vi "Write Wfm.vi"(8 "error in (no error)":errorcluster, 10 "waveform":waveform(dbl)[][](array[waveform]), 11 "[M] TDMS Save in":refnum<class "[M] TDMS Save.lvclass">) -> (0 "error out":errorcluster, 3 "[M] TDMS Save out":refnum<class "[M] TDMS Save.lvclass">)   [LabVIEW 2023, in "[M] TDMS Save.lvlib" / "[M] TDMS Save.lvclass"]
uses:
  [M] TDMS Save.lvclass
  [M] TDMS Save.lvclass/[M] TDMS Save.ctl
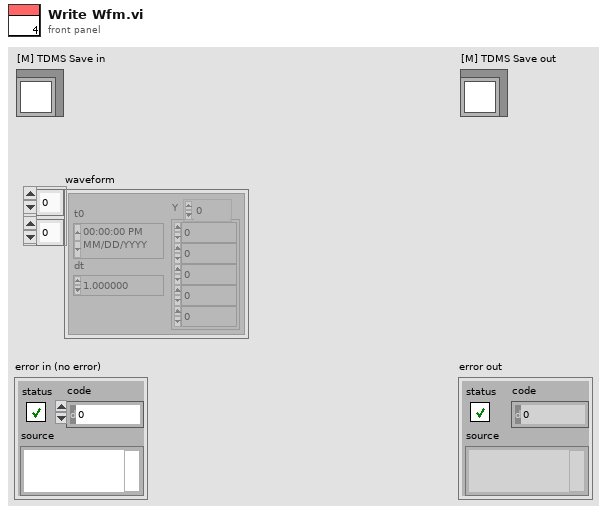
[diagram p1: front panel]
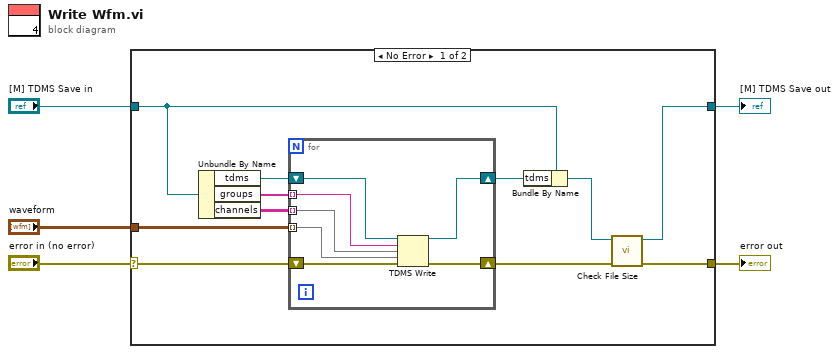
[diagram p0: block diagram]
diagram:
  n1 = case shown="No Error" "error in (no error)" {
    selector: "error in (no error)" -> [w14 w25]
    tunnel: [w8 w25] -> w4
    tunnel: [w6 w24] -> w2
    tunnel: "[M] TDMS Save in" -> [w13 w24]
    tunnel: "waveform" -> [w15 _]
    frame No Error {
      n2 = Unbundle By Name(w13) -> ("tdms"=w16:refnum<k34>, "groups"=w11:string[], "channels"=w10:string[][])
      n3 = for {
        shift-right: [w20] -> w12
        shift-left: w16 -> [w21]
        tunnel: w15 -> [w22] mode=indexing
        shift-right: [w19] -> w9
        shift-left: w14 -> [w23]
        tunnel: w11 -> [w17] mode=indexing
        tunnel: w10 -> [w18] mode=indexing
        n4 = TDMS Write(0:w21, 5:w17, 7:w18, 9:w22, 11:w23) -> (4:w20:refnum<k34>, 15:w19:errorcluster)  [unwired: 1 in, 2 out]
      }
      n5 = Bundle By Name(cluster=w13, "tdms"=w12) -> (w7:refnum<class "[M] TDMS Save.lvclass">)
      n6 = call "Check File Size.vi"("error in (no error)"=w9, "[M] TDMS Save in"=w7) -> ("error out"=w8:errorcluster, "[M] TDMS Save out"=w6:refnum<class "[M] TDMS Save.lvclass">)  [unwired: 8 in]
    }
    frame Error {
    }
  }
  "error out" <- w4
  "[M] TDMS Save out" <- w2
